vi "Script New Event.vi"(0 "LibraryPath":path, 1 "Project":refnum<vi>, 5 "Event Type":T1, 7 "Event Name":string, 11 "error in (no error)":errorcluster) -> (4 "LibraryPathOut":path, 15 "error out":errorcluster)   [LabVIEW 2014, in "DQMH_API.lvclass"]
uses:
  <resource>/Framework/Providers/Open_GDS/UML/DQMH_API_class/DQMH_API.lvclass
  project/Delacor/DQMH/_DQMH New Event/Event Type--enum.ctl
  project/Delacor/DQMH/_DQMH New Event/DQMH New Event.lvlib
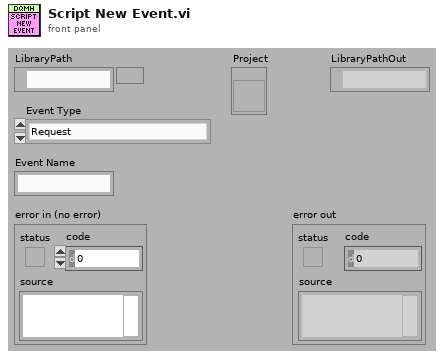
[diagram p1: front panel]
types:
  T1 = typedef "DQMH New Event.lvlib/Event Type--enum.ctl" = enum16{"Request", "Broadcast", "Request and Wait for Reply", "Round Trip"}
  T2 = typedef "DQMH_API.lvclass/ObjectAttributes.ctl" = cluster{"Get Module Type Info":refnum<vi>, "Script New Module":refnum<vi>, "Script New Event":refnum<vi>}
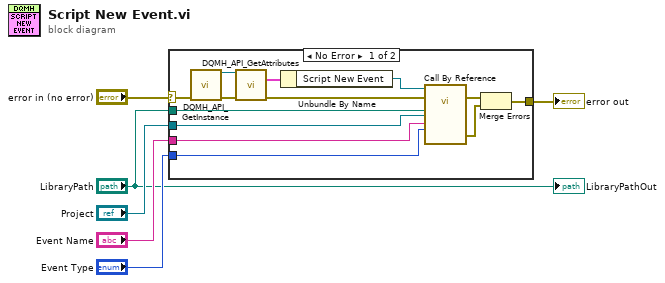
[diagram p0: block diagram]
diagram:
  n1 = case shown="No Error" "error in (no error)" {
    selector: "error in (no error)" -> [w17 w20]
    tunnel: [w13 w20] -> w5
    tunnel: "Event Name" -> [w11 _]
    tunnel: "Event Type" -> [w10 _]
    tunnel: "Project" -> [w9 _]
    tunnel: "LibraryPath" -> [w8 _]
    frame No Error {
      n2 = call <resource>:"DQMH_API_GetInstance.vi"("error in (no error)"=w17) -> ("reference out"=w18:refnum<class "DQMH_API.lvclass">, "error out"=w16:errorcluster)  [unwired: 10 in, 3 out]
      n3 = call <resource>:"DQMH_API_GetAttributes.vi"("reference in"=w18, "error in (no error)"=w16) -> ("Data"=w19:T2, "error out"=w15:errorcluster)  [unwired: 10 in, 2 out]
      n4 = Unbundle By Name(w19) -> ("Script New Event"=w12:refnum<vi>)
      n5 = call-by-ref "?"(reference=w12, error in=w15, "LibraryPath"=w8, "Project"=w9, "Event Name"=w11, "Event Type"=w10) -> (error out=w14:errorcluster, 15:"error out"=w7:errorcluster)  [unwired: 11 in, 1 out]
      n6 = Merge Errors(w14, w7) -> (w13:errorcluster)
    }
    frame Error {
    }
  }
  "error out" <- w5
  "LibraryPathOut" <- "LibraryPath"
